vi "DB Request UI List.vi"(0 "Database in":refnum<queue>, 1 "UI List Type":T3, 2 "UI Device Type":T2, 3 "Measurement Role Selection":T1, 4 "Identifier":i32, 5 "error in (no error)":errorcluster) -> (14 "Database out":refnum<queue>, 15 "Results":string[][](array[string]), 19 "error out":errorcluster)   [LabVIEW 2026, in "Settings.lvlib"]
uses:
  Settings/Settings.lvlib
  support/Architecture/Message Queue/Message Cluster.ctl
  controls/UI/UI List Type.ctl
  controls/UI/UI Device Type.ctl
  controls/UI/Measurement Role Selection.ctl
  controls/Messaging Payloads/DB Query Request Payload.ctl
  support/Architecture/Message Queue/Enqueue Message (Single).vi
  support/Architecture/Message Queue/Message Queue.lvlib
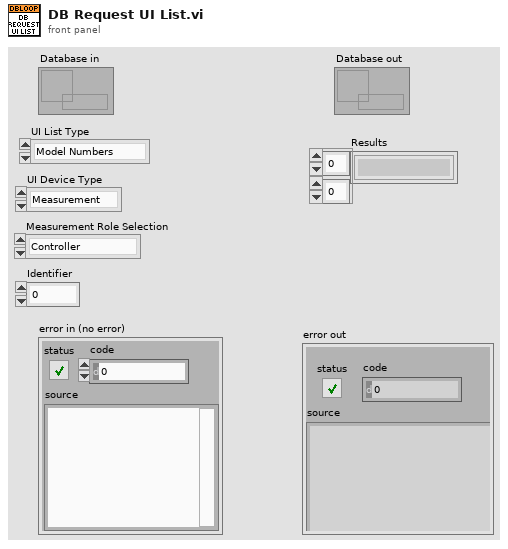
[diagram p1: front panel]
types:
  T1 = typedef "Settings.lvlib/Measurement Role Selection.ctl" = enum16{"Controller", "Reference", "UUT", "All"}
  T2 = typedef "Settings.lvlib/UI Device Type.ctl" = enum16{"Measurement", "Controller"}
  T3 = typedef "UI List Type.ctl" = enum16{"Model Numbers", "Serial Numbers", "Operators", "Calibration Points", "Start Run Times"}
  T4 = typedef "DB Query Request Payload.ctl" = cluster{"1D Notifier":refnum<notifier>, "UI List Type":T3, "UI Device Type":T2, "Identifier":i32, "2D Notifier":refnum<notifier>, "Measurement Role Selection":T1}
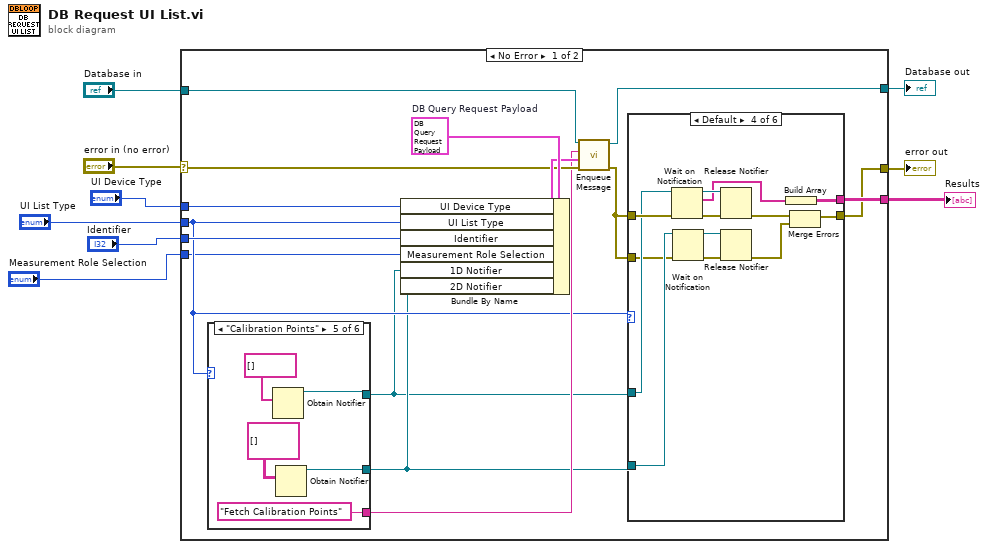
[diagram p0: block diagram]
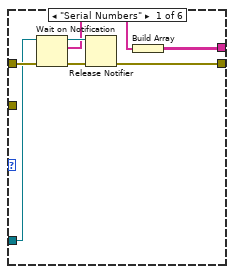
[diagram p2: hidden frame]
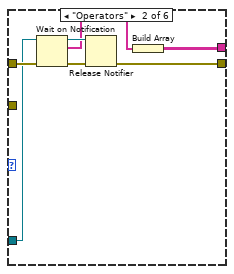
[diagram p3: hidden frame]
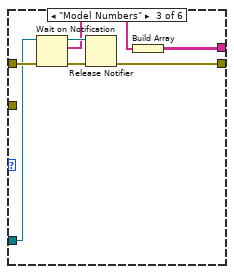
[diagram p4: hidden frame]
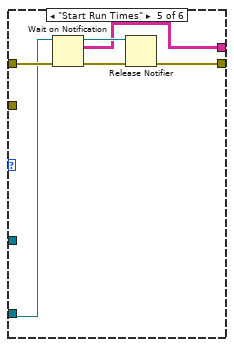
[diagram p5: hidden frame]
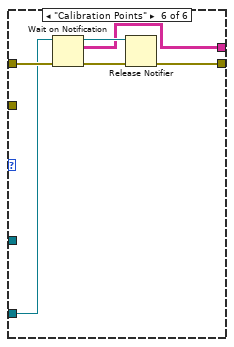
[diagram p6: hidden frame]
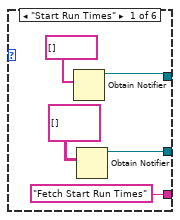
[diagram p7: hidden frame]
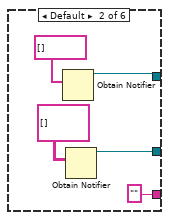
[diagram p8: hidden frame]
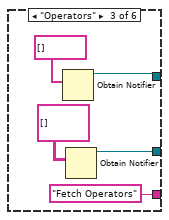
[diagram p9: hidden frame]
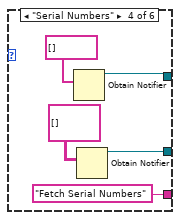
[diagram p10: hidden frame]
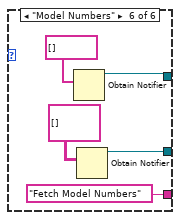
[diagram p11: hidden frame]
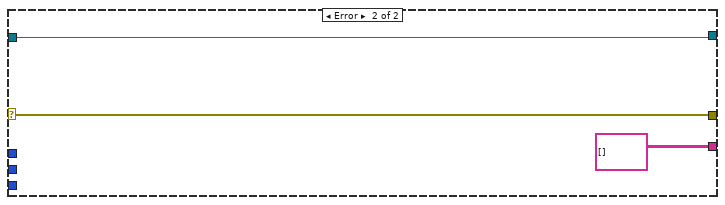
[diagram p12: hidden frame]
diagram:
  n1 = case shown="No Error" "error in (no error)" {
    selector: "error in (no error)" -> [w17 w102]
    tunnel: [w24 string[][] []] -> w2
    tunnel: [w23 w103] -> w9
    tunnel: "Database in" -> [w22 w103]
    tunnel: [w13 w102] -> w7
    tunnel: "UI List Type" -> [w15 _]
    tunnel: "UI Device Type" -> [w19 _]
    tunnel: "Identifier" -> [w18 _]
    tunnel: "Measurement Role Selection" -> [w10 _]
    frame No Error {
      w21 = T4 {"1D Notifier"=refnum, "UI List Type"=enum."Model Numbers", "UI Device Type"=enum."Measurement", "Identifier"=0, "2D Notifier"=refnum, "Measurement Role Selection"=enum."Controller"}  # DB Query Request Payload
      n2 = case shown="\"Calibration Points\"" w15 {
        tunnel: ["Fetch Start Run Times" ("Message") "" ("Message") "Fetch Operators" ("Message") "Fetch Serial Numbers" ("Message") "Fetch Calibration Points" ("Message") "Fetch Model Numbers" ("Message")] -> w16
        tunnel: [w71 w76 w81 w86 w91 w96] -> w11
        tunnel: [w73 w78 w83 w88 w93 w98] -> w14
        frame "Start Run Times" {
          n3 = Obtain Notifier(notification data type=string[] []) -> (notifier out=w71:refnum<notifier>)  [unwired: 3 in, 2 out]
          n4 = Obtain Notifier(notification data type=string[][] []) -> (notifier out=w73:refnum<notifier>)  [unwired: 3 in, 2 out]
        }
        frame Default {
          n5 = Obtain Notifier(notification data type=string[] []) -> (notifier out=w76:refnum<notifier>)  [unwired: 3 in, 2 out]
          n6 = Obtain Notifier(notification data type=string[][] []) -> (notifier out=w78:refnum<notifier>)  [unwired: 3 in, 2 out]
        }
        frame "Operators" {
          n7 = Obtain Notifier(notification data type=string[] []) -> (notifier out=w81:refnum<notifier>)  [unwired: 3 in, 2 out]
          n8 = Obtain Notifier(notification data type=string[][] []) -> (notifier out=w83:refnum<notifier>)  [unwired: 3 in, 2 out]
        }
        frame "Serial Numbers" {
          n9 = Obtain Notifier(notification data type=string[] []) -> (notifier out=w86:refnum<notifier>)  [unwired: 3 in, 2 out]
          n10 = Obtain Notifier(notification data type=string[][] []) -> (notifier out=w88:refnum<notifier>)  [unwired: 3 in, 2 out]
        }
        frame "Calibration Points" {
          n11 = Obtain Notifier(notification data type=string[] []) -> (notifier out=w91:refnum<notifier>)  [unwired: 3 in, 2 out]
          n12 = Obtain Notifier(notification data type=string[][] []) -> (notifier out=w93:refnum<notifier>)  [unwired: 3 in, 2 out]
        }
        frame "Model Numbers" {
          n13 = Obtain Notifier(notification data type=string[] []) -> (notifier out=w96:refnum<notifier>)  [unwired: 3 in, 2 out]
          n14 = Obtain Notifier(notification data type=string[][] []) -> (notifier out=w98:refnum<notifier>)  [unwired: 3 in, 2 out]
        }
      }
      n15 = Bundle By Name(cluster=w21, "UI Device Type"=w19, "UI List Type"=w15, "Identifier"=w18, "Measurement Role Selection"=w10, "1D Notifier"=w11, "2D Notifier"=w14) -> (w20:T4)
      n16 = call-poly "Enqueue Message.vi"("error in (no error)"=w17, "Message Data"=w20, "Message"=w16, "Message Queue"=w22) -> ("error out"=w12:errorcluster, "dup Message Queue"=w23:refnum<queue>)  [unwired: 6 in]
      n17 = case shown="Default" w15 {
        tunnel: [w29 w36 w43 w56 w59 w65] -> w24
        tunnel: [w27 w34 w41 w46 w60 w66] -> w13
        tunnel: w12 -> [w31 w38 w45 w58 w64 w70]
        tunnel: w11 -> [w30 w37 w44 w57 _ _]
        tunnel: w14 -> [_ _ _ w51 w63 w69]
        tunnel: w12 -> [_ _ _ w49 _ _]
        frame "Serial Numbers" {
          n18 = Wait on Notification(notifier=w30, error in (no error)=w31) -> (notifier out=w26:refnum<notifier>, notification=w25:string[], error out=w28:errorcluster)  [unwired: 2 in, 1 out]
          n19 = Release Notifier(notifier=w26, error in (no error)=w28) -> (error out=w27:errorcluster)  [unwired: 1 in, 2 out]
          n20 = Build Array(w25) -> (w29:string[][])
        }
        frame "Operators" {
          n21 = Wait on Notification(notifier=w37, error in (no error)=w38) -> (notifier out=w33:refnum<notifier>, notification=w32:string[], error out=w35:errorcluster)  [unwired: 2 in, 1 out]
          n22 = Release Notifier(notifier=w33, error in (no error)=w35) -> (error out=w34:errorcluster)  [unwired: 1 in, 2 out]
          n23 = Build Array(w32) -> (w36:string[][])
        }
        frame "Model Numbers" {
          n24 = Wait on Notification(notifier=w44, error in (no error)=w45) -> (notifier out=w40:refnum<notifier>, notification=w39:string[], error out=w42:errorcluster)  [unwired: 2 in, 1 out]
          n25 = Release Notifier(notifier=w40, error in (no error)=w42) -> (error out=w41:errorcluster)  [unwired: 1 in, 2 out]
          n26 = Build Array(w39) -> (w43:string[][])
        }
        frame Default {
          n27 = Wait on Notification(notifier=w57, error in (no error)=w58) -> (notifier out=w54:refnum<notifier>, notification=w53:string[], error out=w55:errorcluster)  [unwired: 2 in, 1 out]
          n28 = Wait on Notification(notifier=w51, error in (no error)=w49) -> (notifier out=w52:refnum<notifier>, error out=w50:errorcluster)  [unwired: 2 in, 2 out]
          n29 = Release Notifier(notifier=w54, error in (no error)=w55) -> (error out=w47:errorcluster)  [unwired: 1 in, 2 out]
          n30 = Release Notifier(notifier=w52, error in (no error)=w50) -> (error out=w48:errorcluster)  [unwired: 1 in, 2 out]
          n31 = Build Array(w53) -> (w56:string[][])
          n32 = Merge Errors(w47, w48) -> (w46:errorcluster)
        }
        frame "Start Run Times" {
          n33 = Wait on Notification(notifier=w63, error in (no error)=w64) -> (notifier out=w62:refnum<notifier>, notification=w59:string[][], error out=w61:errorcluster)  [unwired: 2 in, 1 out]
          n34 = Release Notifier(notifier=w62, error in (no error)=w61) -> (error out=w60:errorcluster)  [unwired: 1 in, 2 out]
        }
        frame "Calibration Points" {
          n35 = Wait on Notification(notifier=w69, error in (no error)=w70) -> (notifier out=w68:refnum<notifier>, notification=w65:string[][], error out=w67:errorcluster)  [unwired: 2 in, 1 out]
          n36 = Release Notifier(notifier=w68, error in (no error)=w67) -> (error out=w66:errorcluster)  [unwired: 1 in, 2 out]
        }
      }
    }
    frame Error {
    }
  }
  "Database out" <- w9
  "error out" <- w7
  "Results" <- w2
